vi "Agilent U2000 Series Range Test Characteristic.vi"() -> ()   [LabVIEW 2018]
doc: "This example shows how to configure a range and check that the acquired measurements are within that range using the VIs of the driver.\n\nNote:\nThis example is applicable for U2021/2XA only."
uses:
  Agilent U2000 Series.lvlib
panel:
  out "Out of Range":bool
  in  "Lower Limit (-90.0 dBm)":dbl=-90.0 format="%#.6g"
  in  "Upper Limit (90.0 dBm)":dbl=90.0 format="%#.6g"
  in  "Timeout (10000 ms)":u32=10000
  out "Measurement":dbl
  in  "VISA resource name":refnum<visa-resource-name>
  # "(c) 2011-2015 National Instruments.  ALL RIGHTS RESERVED."
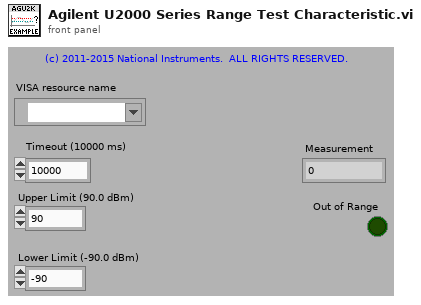
[diagram p1: front panel]
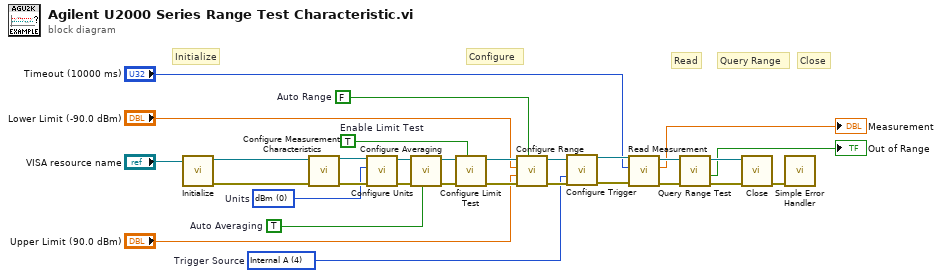
[diagram p0: block diagram]
diagram:
  w1 = 0 items=["dBm", "Watts"]  # Units
  w8 = TRUE  # Enable Limit Test
  w10 = 4 items=["Bus", "External", "Hold", "Immediate", "Internal A"]  # Trigger Source
  w3 = TRUE  # Auto Averaging
  w9 = FALSE  # Auto Range
  # "Query Range"
  # "Close"
  # "Read"
  # "Configure"
  # "Initialize"
  n1 = call "Initialize.vi"("VISA resource name"="VISA resource name") -> ("error out"=w4:errorcluster, "VISA resource name out"=w5:refnum<visa-resource-name>)  [unwired: 3 in, 6 out]
  n2 = call "Configure Measurement Characteristics.vi"("VISA resource name"=w5, "error in (no error)"=w4) -> ("VISA resource name out"=w28:refnum<visa-resource-name>, "error out"=w29:errorcluster)  [unwired: 12 in]
  n3 = call "Configure Units.vi"("error in (no error)"=w29, "Units (0: dBm)"=w1, "VISA resource name"=w28) -> ("error out"=w27:errorcluster, "VISA resource name out"=w26:refnum<visa-resource-name>)  [unwired: 1 in, 6 out]
  n4 = call "Configure Averaging.vi"("Auto Averaging (T: Enable)"=w3, "error in (no error)"=w27, "VISA resource name"=w26) -> ("error out"=w25:errorcluster, "VISA resource name out"=w24:refnum<visa-resource-name>)  [unwired: 7 in]
  n5 = call "Configure Limit Test.vi"("Limit Test (T: Enable)"=w8, "error in (no error)"=w25, "VISA resource name"=w24) -> ("error out"=w23:errorcluster, "VISA resource name out"=w22:refnum<visa-resource-name>)  [unwired: 2 in, 5 out]
  n6 = call "Configure Range.vi"("Auto Range (T: Enable)"=w9, "error in (no error)"=w23, "Upper Limit (90 dBm)"="Upper Limit (90.0 dBm)", "Lower Limit (-90 dBm)"="Lower Limit (-90.0 dBm)", "VISA resource name"=w22) -> ("error out"=w11:errorcluster, "VISA resource name out"=w2:refnum<visa-resource-name>)  [unwired: 5 in]
  n7 = call "Configure Trigger.vi"("VISA resource name"=w2, "Trigger Source (3: Immediate)"=w10, "error in (no error)"=w11) -> ("VISA resource name out"=w20:refnum<visa-resource-name>, "error out"=w21:errorcluster)  [unwired: 5 in, 6 out]
  n8 = call "Read Measurement.vi"("error in (no error)"=w21, "Timeout (10000 ms)"="Timeout (10000 ms)", "VISA resource name"=w20) -> ("error out"=w19:errorcluster, "Measurement"=→"Measurement":dbl, "VISA resource name out"=w18:refnum<visa-resource-name>)  [unwired: 6 out]
  n9 = call "Query Range Test.vi"("error in (no error)"=w19, "VISA resource name"=w18) -> ("error out"=w15:errorcluster, "Limit Failure?"=→"Out of Range":bool, "VISA resource name out"=w16:refnum<visa-resource-name>)  [unwired: 1 in, 6 out]
  n10 = call "Close.vi"("error in (no error)"=w15, "VISA resource name"=w16) -> ("error out"=w17:errorcluster)  [unwired: 9 out]
  n11 = call <vilib>:"Simple Error Handler.vi"("error in (no error)"=w17) -> ()  [unwired: 1 in, 8 out]
